vi "Write Message (read).vi"(6 "ID (Read)":string, 8 "error in (no error)":errorcluster, 9 "Data (Read)":variant, 10 "Command (Read)":string, 11 "RemoteControl in":refnum<class "RemoteControl.lvclass">) -> (0 "error out":errorcluster, 3 "RemoteControl out":refnum<class "RemoteControl.lvclass">)   [LabVIEW 2019, in "RemoteControl.lvclass"]
uses:
  RemoteControl.lvclass
  RemoteControl.lvclass/RemoteControl.ctl
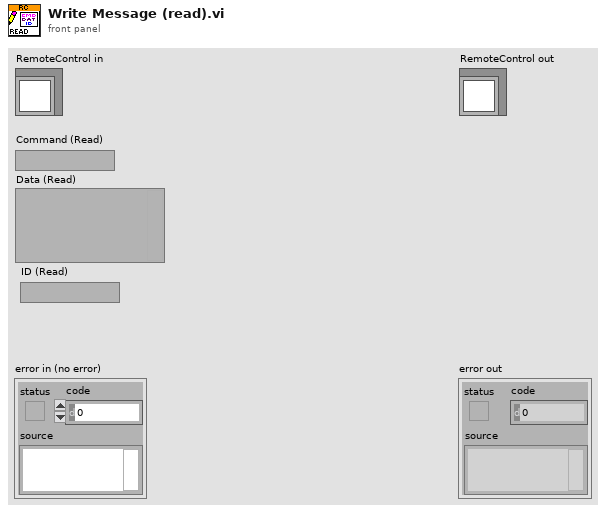
[diagram p1: front panel]
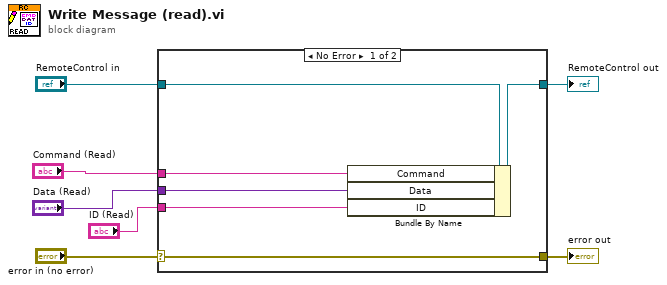
[diagram p0: block diagram]
diagram:
  n1 = case shown="No Error" "error in (no error)" {
    selector: "error in (no error)" -> [w13 w14]
    tunnel: [w13 w14] -> w6
    tunnel: [w11 w15] -> w4
    tunnel: "RemoteControl in" -> [w12 w15]
    tunnel: "Command (Read)" -> [w10 _]
    tunnel: "Data (Read)" -> [w9 _]
    tunnel: "ID (Read)" -> [w8 _]
    frame No Error {
      n2 = Bundle By Name(cluster=w12, "Command"=w10, "Data"=w9, "ID"=w8) -> (w11:refnum<class "RemoteControl.lvclass">)
    }
    frame Error {
    }
  }
  "error out" <- w6
  "RemoteControl out" <- w4
